vi "CreatePrivateEvents.vi"(8 "error in (no error)":errorcluster, 11 "RemoteControl":refnum<class "LockinRemoteControl.lvclass">) -> (0 "error out":errorcluster, 3 "RemoteControl out":refnum<class "LockinRemoteControl.lvclass">)   [LabVIEW 2016, in "LockinRemoteControl.lvclass"]
doc: "---------------------------------------------------------------\nJKI State Machine Objects™\nhttp://jki.net/state-machine-objects/\nCopyright (C) 2005-2015, JKI <info@jki.net>\nALL RIGHTS RESERVEDJKI State Machine Objects (SMO) 1.0.0.4\nJKI - JKI\nCopyright (c) 2015, JKI"
uses:
  LockinRemoteControl.lvclass
  Typedefs/PrivateEvents--LockinRemoteControl.setAllowedRemoteAddress.ctl
  Typedefs/PrivateEvents--LockinRemoteControl.setAO.ctl
  Typedefs/PrivateEvents--LockinRemoteControl.setAI.ctl
  Typedefs/PrivateEvents--LockinRemoteControl.setResults.ctl
  Typedefs/PrivateEvents--LockinRemoteControl.setTrigger.ctl
  Typedefs/PrivateEvents--LockinRemoteControl.setAOconfig.ctl
  Typedefs/AO-cluster.ctl
  Typedefs/AO_Amp-array.ctl
  Typedefs/AO_DC-array.ctl
  Typedefs/AO_f-array.ctl
  Typedefs/AO_phi-array.ctl
  Typedefs/Function-array.ctl
  Typedefs/Function-enum.ctl
  Typedefs/PrivateEvents--LockinRemoteControl.setREFconfig.ctl
  Typedefs/REF-cluster.ctl
  Typedefs/REF_f-array.ctl
  Typedefs/REF_phi-array.ctl
  Typedefs/PrivateEvents--LockinRemoteControl.setReset.ctl
  Typedefs/PrivateEvents--LockinRemoteControl.setIVmode.ctl
  Typedefs/PrivateEvents--LockinRemoteControl.setREFfilterconfig.ctl
  LockinRemoteControl.lvclass/LockinRemoteControl.ctl
  <vilib>/JKI/JKI SMO/SMO/SMO.lvclass
panel:
  # "For instructions on how to use the JKI State Machine Objects, examples and video tutorials, visit:\nhttp://jki.net/state-machine-objects/\n\nJKI State Machine Objects™\nhttp://jki.net/state-machine-objects/\nCopyright (C) 2005-2015, JKI <info@jki.net>\nALL RIGHTS RESERVED"
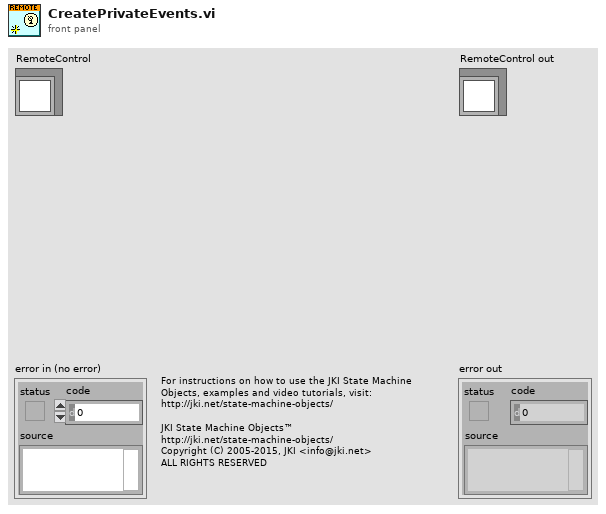
[diagram p1: front panel]
types:
  T1 = typedef "LockinRemoteControl.lvclass/PrivateEvents--LockinRemoteControl.setREFfilterconfig.ctl" = cluster{"TC (s)":dbl, "order":i32}
  T2 = typedef "LockinRemoteControl.lvclass/PrivateEvents--LockinRemoteControl.setIVmode.ctl" = bool
  T3 = typedef "LockinRemoteControl.lvclass/PrivateEvents--LockinRemoteControl.setReset.ctl" = bool
  T4 = typedef "LockinRemoteControl.lvclass/PrivateEvents--LockinRemoteControl.setREFconfig.ctl" = cluster{"Channels: Lockin":T5}
  T5 = typedef "REF-cluster.ctl" = cluster{"REF f (Hz)":T6, "REF phi (°)":T7}
  T6 = typedef "REF_f-array.ctl" = dbl[]
  T7 = typedef "REF_phi-array.ctl" = dbl[]
  T8 = typedef "LockinRemoteControl.lvclass/PrivateEvents--LockinRemoteControl.setAOconfig.ctl" = cluster{"Channels: AO":T9}
  T9 = typedef "AO-cluster.ctl" = cluster{"AO amp (V)":T10, "AO DC (V)":T11, "AO f (Hz)":T12, "AO phi (°)":T13, "function":T14, "I+":bool[]}
  T10 = typedef "AO_Amp-array.ctl" = dbl[]
  T11 = typedef "AO_DC-array.ctl" = dbl[]
  T12 = typedef "AO_f-array.ctl" = dbl[]
  T13 = typedef "AO_phi-array.ctl" = dbl[]
  T14 = typedef "Function-array.ctl" = T15[]
  T15 = typedef "Function-enum.ctl" = enum16{"Sine", "Triangle", "Square", "Sawtooth"}
  T16 = typedef "LockinRemoteControl.lvclass/PrivateEvents--LockinRemoteControl.setTrigger.ctl" = bool
  T17 = typedef "LockinRemoteControl.lvclass/PrivateEvents--LockinRemoteControl.setResults.ctl" = cluster{"Time Stamp":timestamp, "setResults":dbl[][]}
  T18 = typedef "LockinRemoteControl.lvclass/PrivateEvents--LockinRemoteControl.setAI.ctl" = waveform(dbl)[]
  T19 = typedef "LockinRemoteControl.lvclass/PrivateEvents--LockinRemoteControl.setAO.ctl" = waveform(dbl)[]
  T20 = typedef "LockinRemoteControl.lvclass/PrivateEvents--LockinRemoteControl.setAllowedRemoteAddress.ctl" = string
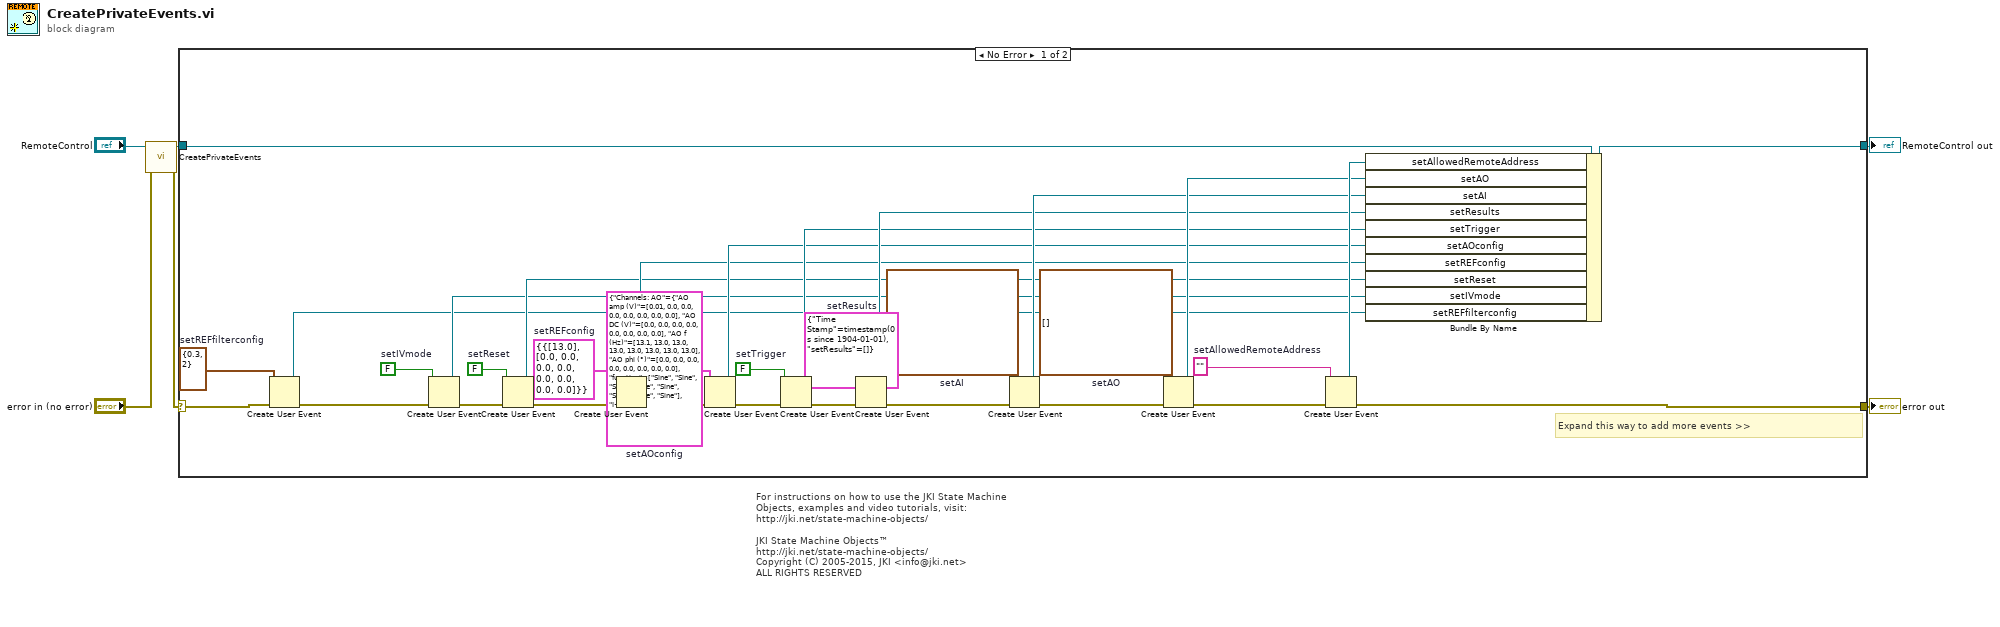
[diagram p0: block diagram]
diagram:
  # "For instructions on how to use the JKI State Machine Objects, examples and video tutorials, visit:\nhttp://jki.net/state-machine-objects/\n\nJKI State Machine Objects™\nhttp://jki.net/state-machine-objects/\nCopyright (C) 2005-2015, JKI <info@jki.net>\nALL RIGHTS RESERVED"
  n1 = call-parent "CreatePrivateEvents.vi"("error in (no error)"="error in (no error)", "SMO"="RemoteControl") -> ("error out"=w1:errorcluster, "SMO out"=w3:refnum<class "LockinRemoteControl.lvclass">)  [unwired: 8 in]
  n2 = case shown="No Error" w1 {
    selector: w1 -> [w10 w41]
    tunnel: [w37 w41] -> w5
    tunnel: [w38 w40] -> w6
    tunnel: w3 -> [w39 w40]
    frame No Error {
      w8 = T1 {"TC (s)"=0.3, "order"=2}  # setREFfilterconfig
      w12 = T2 FALSE  # setIVmode
      w15 = T3 FALSE  # setReset
      w18 = T4 {"Channels: Lockin"={"REF f (Hz)"=[13.0], "REF phi (°)"=[0.0, 0.0, 0.0, 0.0, 0.0, 0.0, 0.0, 0.0]}}  # setREFconfig
      w21 = T8 {"Channels: AO"={"AO amp (V)"=[0.01, 0.0, 0.0, 0.0, 0.0, 0.0, 0.0, 0.0], "AO DC (V)"=[0.0, 0.0, 0.0, 0.0, 0.0, 0.0, 0.0, 0.0], "AO f (Hz)"=[13.1, 13.0, 13.0, 13.0, 13.0, 13.0, 13.0, 13.0], "AO phi (°)"=[0.0, 0.0, 0.0, 0.0, 0.0, 0.0, 0.0, 0.0], "function"=[enum."Sine", enum."Sine", enum."Sine", enum."Sine", enum."Sine", enum."Sine", enum."Sine", enum."Sine"], "I+"=[]}}  # setAOconfig
      w24 = T16 FALSE  # setTrigger
      w27 = T17 {"Time Stamp"=timestamp(0 s since 1904-01-01), "setResults"=[]}  # setResults
      w30 = T18 []  # setAI
      w33 = T19 []  # setAO
      w36 = T20 ""  # setAllowedRemoteAddress
      # "Expand this way to add more events >>"
      n3 = Create User Event(user event datatype=w8, error in=w10) -> (user event=w7:refnum<user-event>, error out=w9:errorcluster)
      n4 = Create User Event(user event datatype=w12, error in=w9) -> (user event=w11:refnum<user-event>, error out=w13:errorcluster)
      n5 = Create User Event(user event datatype=w15, error in=w13) -> (user event=w14:refnum<user-event>, error out=w16:errorcluster)
      n6 = Create User Event(user event datatype=w18, error in=w16) -> (user event=w17:refnum<user-event>, error out=w19:errorcluster)
      n7 = Create User Event(user event datatype=w21, error in=w19) -> (user event=w20:refnum<user-event>, error out=w22:errorcluster)
      n8 = Create User Event(user event datatype=w24, error in=w22) -> (user event=w23:refnum<user-event>, error out=w25:errorcluster)
      n9 = Create User Event(user event datatype=w27, error in=w25) -> (user event=w26:refnum<user-event>, error out=w28:errorcluster)
      n10 = Create User Event(user event datatype=w30, error in=w28) -> (user event=w29:refnum<user-event>, error out=w31:errorcluster)
      n11 = Create User Event(user event datatype=w33, error in=w31) -> (user event=w32:refnum<user-event>, error out=w34:errorcluster)
      n12 = Create User Event(user event datatype=w36, error in=w34) -> (user event=w35:refnum<user-event>, error out=w37:errorcluster)
      n13 = Bundle By Name(cluster=w39, "setAllowedRemoteAddress"=w35, "setAO"=w32, "setAI"=w29, "setResults"=w26, "setTrigger"=w23, "setAOconfig"=w20, "setREFconfig"=w17, "setReset"=w14, "setIVmode"=w11, "setREFfilterconfig"=w7) -> (w38:refnum<class "LockinRemoteControl.lvclass">)
    }
    frame Error {
    }
  }
  "error out" <- w5
  "RemoteControl out" <- w6
